vi "GetValue(Generic).vi"(7 "error in (no error)":errorcluster, 11 "TestClass in":refnum<class>) -> (2 "Value":i32, 3 "TestClass out":refnum<class "TestClass.lvclass">, 5 "error out":errorcluster)   [LabVIEW 2009]
doc: "Provides a Get method for the TestClass\nIncludes a downcast from the standard LabVIEW object"
uses:
  TestClass.lvclass
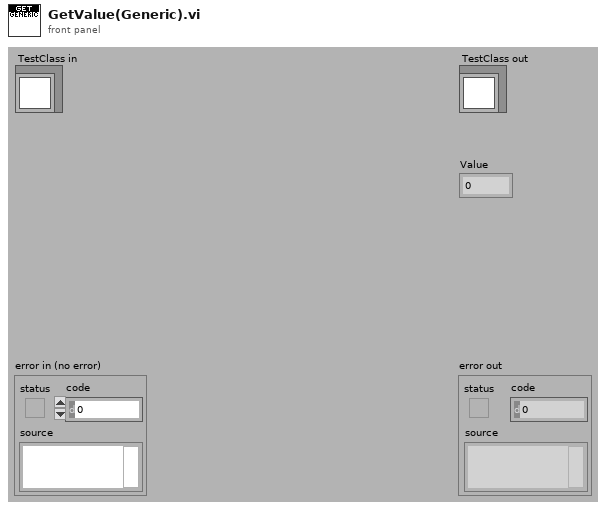
[diagram p1: front panel]
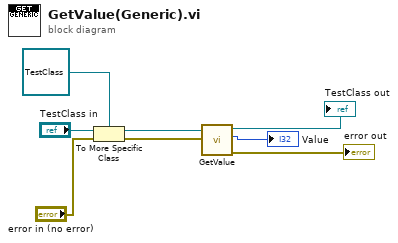
[diagram p0: block diagram]
diagram:
  n1 = To More Specific Class(target class=refnum<class "TestClass.lvclass"> refnum ("TestClass out"), reference="TestClass in", error in="error in (no error)") -> (specific class reference=w5:refnum<class "TestClass.lvclass">, error out=w1:errorcluster)
  n2 = call-dynamic "GetValue.vi"("error in (no error)"=w1, "TestClass in"=w5) -> ("error out"=→"error out":errorcluster, "Value"=→"Value":i32, "TestClass out"=→"TestClass out":refnum<class "TestClass.lvclass">)  [unwired: 7 in]
